vi "GetUsersForListBox.vi"(8 "error in (no error)":errorcluster) -> (0 "error out":errorcluster, 3 "User Name List Box":string[][](array[string]))   [LabVIEW 2017]
doc: "Use this template to build a VI to use as a subVI."
uses:
  DatabaseContollerGFVenum.ctl
  <vilib>/addons/Database/_DB Variant To Data/Database Variant To Data.xnode
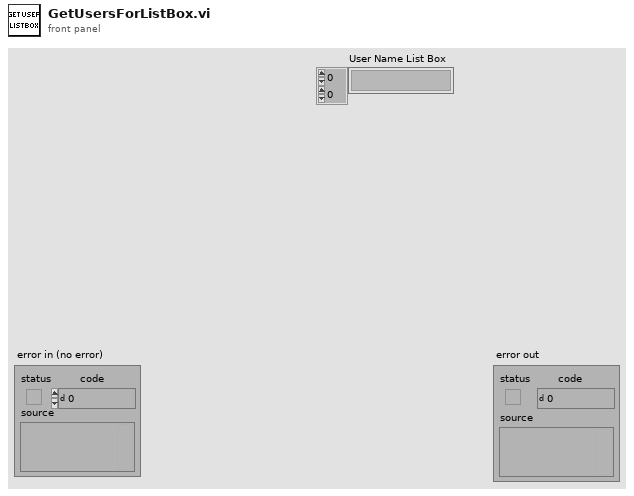
[diagram p1: front panel]
types:
  T1 = typedef "DatabaseContollerGFVenum.ctl" = enum16{"WriteNewUserData!", "Init and Open Database!", "GetAllObjectives!", "GetObjectivesForListBox", "UpdateUserData!", "GetUserData!", "GetUsersAllTable!", "GetTimeDifferencebetweenLastTwoMeasurements!", "Get next Journal Number!", "WriteInJournalTable", "GetNewMeas_dataIndex", "UpdateWithSpectrometerData", "UpdateWithMicroscopeData", "UpdateWithMapScriptData", "UpdateWithmainUIData", "Get Objective Microns/Pixels", "Get User Name!", "Get Next User ID!", "Get Active Users Names!", "Get User Picture!", "Get User Phone Number!", "Get Setup Names!", "Get Active Microscope Objectives!", "Get Experiment Number!", "Get Sample Types!", "Write meas_conf Table", "Write meas_data Table", "GetListOfIndices", "Get Objective Index", "Get last X Journal Entries"}
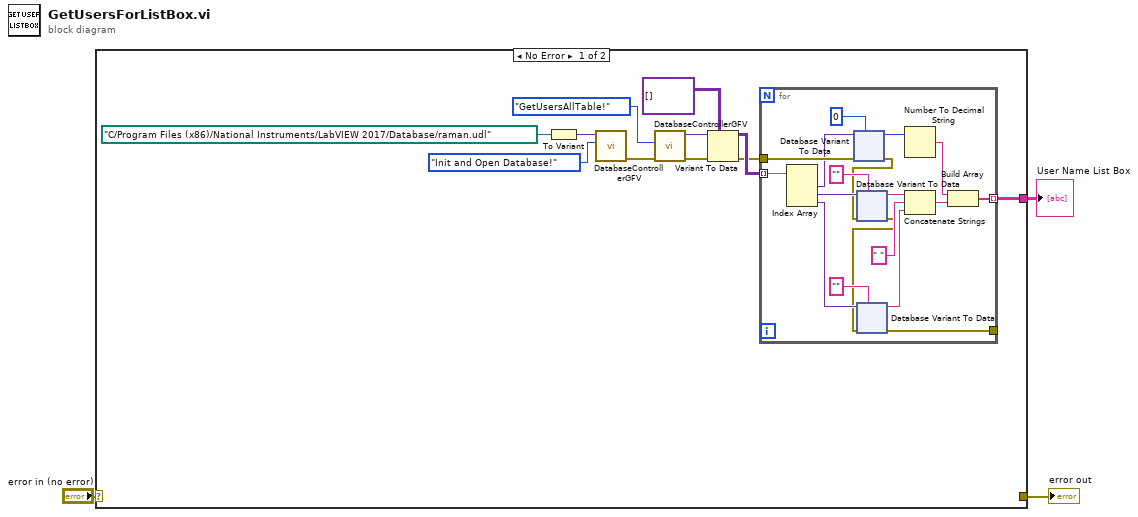
[diagram p0: block diagram]
diagram:
  n1 = case shown="No Error" "error in (no error)" {
    selector: "error in (no error)" -> [_ w129]
    tunnel: [_ w129] -> w2
    tunnel: [w4 _] -> w1
    frame No Error {
      n2 = To Variant(anything=path "C:/Program Files (x86)/National Instruments/LabVIEW 2017/Database/raman.udl" ("connection information")) -> (Variant=w13:variant)
      n3 = call "DatabaseControllerGFV.vi"("Enum"=DatabaseContollerGFVenum."Init and Open Database!", "Data in"=w13) -> ("error out"=w11:errorcluster)  [unwired: 8 in, 1 out]
      n4 = call "DatabaseControllerGFV.vi"("error in (no error)"=w11, "Enum"=DatabaseContollerGFVenum."GetUsersAllTable!") -> ("error out"=w9:errorcluster, "Data Out"=w8:variant)  [unwired: 8 in]
      n5 = Variant To Data(error in=w9, type=variant[][] [] ("data"), Variant=w8) -> (data=w6:variant[][], error out=w5:errorcluster)
      n6 = for {
        tunnel: w6 -> [w31] mode=indexing
        tunnel: w5 -> [w32]
        tunnel: [w20] -> w4 mode=indexing
        tunnel: [w15] -> _
        n7 = Index Array(array=w31) -> (element #1=w30:variant, element #2=w28:variant, element #3=w25:variant)  [unwired: 3 in]
        n8 = xnode "Database Variant To Data"("database variant"=w30, "error in (no error)"=w32, "type"=0) -> ("data"=w23:i32, "error out"=w17:errorcluster)
        n9 = xnode "Database Variant To Data"("database variant"=w28, "error in (no error)"=w17, "type"="") -> ("data"=w19:string, "error out"=w16:errorcluster)
        n10 = xnode "Database Variant To Data"("database variant"=w25, "error in (no error)"=w16, "type"="") -> ("data"=w18:string, "error out"=w15:errorcluster)
        n11 = Number To Decimal String(number=w23) -> (decimal integer string=w22:string)  [unwired: 1 in]
        n12 = Concatenate Strings(w19, " " ("string"), w18) -> (w21:string)
        n13 = Build Array(w22, w21) -> (w20:string[])
      }
    }
    frame Error {
    }
  }
  "error out" <- w2
  "User Name List Box" <- w1
